vi "Heat2D_Solver.vi"(0 "F(t, x, y)":dbl[][][](array[numeric]), 1 "Initial Value":dbl[][](array[numeric]), 5 "k":dbl=1.0, 7 "a":dbl, 9 "Domain":T1={"t"={"initial t"=0.0, "final t"=1.0, "# of t-points"=11}, "x"={"start x"=0.0, "end x"=1.0, "# of x-points"=11}, "y"={"start y"=0.0, "end y"=1.0, "# of y-points"=11}}, 11 "error in (no error)":errorcluster, 12 "Boundary Condition":cluster{"type":T2, "Value":dbl[][]}[](array[cluster]) {"type" items=["Dirichlet", "Neumann"]}) -> (4 "U(t, x, y)":dbl[][][](array[numeric]), 15 "error out":errorcluster)   [LabVIEW 2020, in "NI_PDE.lvlib"]
uses:
  <vilib>/gmath/NI_PDE.lvlib
  <vilib>/gmath/pde.llb/Common/PDE_BC Type.ctl
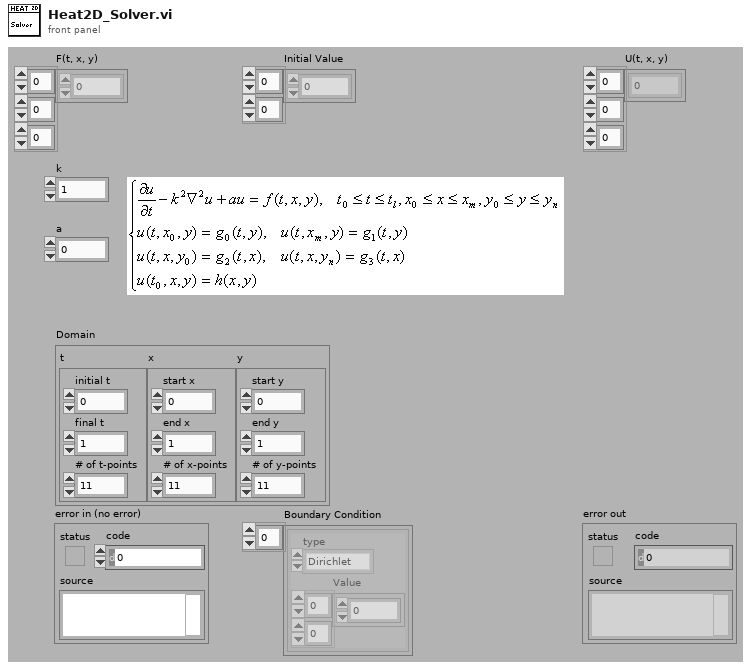
[diagram p1: front panel]
types:
  T1 = cluster{"t":cluster{"initial t":dbl, "final t":dbl, "# of t-points":i32}, "x":cluster{"start x":dbl, "end x":dbl, "# of x-points":i32}, "y":cluster{"start y":dbl, "end y":dbl, "# of y-points":i32}}
  T2 = typedef "NI_PDE.lvlib/PDE_BC Type.ctl" = i32
  T3 = cluster{"rx":dbl, "ry":dbl, "s":dbl, "c":dbl, "deltaT":dbl, "deltaX":dbl, "deltaY":dbl}
  T4 = cluster{"X LU Factor":cluster{"L":dbl[], "U":cluster{"Diagonal":dbl[], "Super Diagonal":dbl[], "2nd Super Diagonal":dbl[]}, "Pivot":i32[]}, "Y LU Factor":cluster{"L":dbl[], "U":cluster{"Diagonal":dbl[], "Super Diagonal":dbl[], "2nd Super Diagonal":dbl[]}, "Pivot":i32[]}, "X Tridiagonal":cluster{"SubDiagonal":dbl[], "MainDiagonal":dbl[], "SuperDiagonal":dbl[]}, "Y Tridiagonal":cluster{"SubDiagonal":dbl[], "MainDiagonal":dbl[], "SuperDiagonal":dbl[]}}
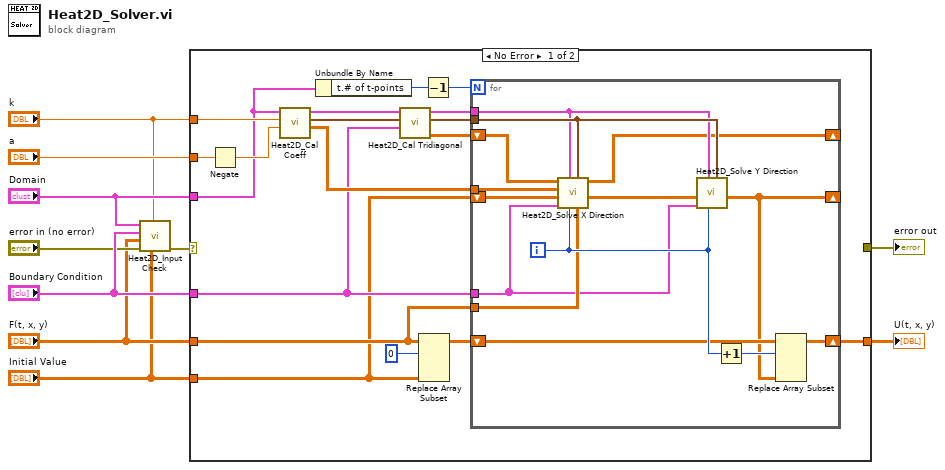
[diagram p0: block diagram]
diagram:
  n1 = call <vilib>:"Heat2D_Input Check.vi"("Initial Value"="Initial Value", "k"="k", "error in (no error)"="error in (no error)", "F(t, x, y)"="F(t, x, y)", "Boundary Condition"="Boundary Condition", "Domain"="Domain") -> ("error out"=w7:errorcluster)  [unwired: 5 out]
  n2 = case shown="No Error" w7 {
    selector: w7 -> [_ w43]
    tunnel: "k" -> [w28 _]
    tunnel: "a" -> [w27 _]
    tunnel: "Initial Value" -> [w11 _]
    tunnel: "Boundary Condition" -> [w12 _]
    tunnel: "F(t, x, y)" -> [w13 _]
    tunnel: "Domain" -> [w14 _]
    tunnel: [_ w43] -> w3
    tunnel: [w20 _] -> w2
    frame No Error {
      n3 = Negate(x=w27) -> (-x=w24:dbl)
      n4 = call <vilib>:"Heat2D_Cal Coeff.vi"("a"=w24, "k"=w28, "Domain"=w14) -> ("Matr_RHS"=w23:dbl[][], "Coefficients"=w17:T3, "Domain Dup"=w26:T1)  [unwired: 6 out]
      n5 = Unbundle By Name(w14) -> ("t.# of t-points"=w16:i32)
      n6 = call <vilib>:"Heat2D_Cal Tridiagonal.vi"("Boundary Condition"=w12, "Coefficients"=w17, "Domain"=w26) -> ("X RHS"=w18:dbl[][], "Coefficients Dup"=w25:T3, "TriDia Cluster"=w19:T4)  [unwired: 1 in, 5 out]
      n7 = Replace Array Subset(array=w13, new element=w11, index (dim 0)=0 ("index (page)")) -> (w22:dbl[][][])  [unwired: 2 in]
      n8 = Decrement(x=w16) -> (x-1=w15:i32)
      n9 = for {
        N: w15 -> [_]
        shift-right: [w29] -> _
        shift-left: w11 -> [w32]
        tunnel: w25 -> [w42]
        tunnel: w12 -> [w31]
        tunnel: w13 -> [w34]
        tunnel: w23 -> [w33]
        shift-right: [w35] -> w20
        shift-left: w22 -> [w36]
        tunnel: w19 -> [w40]
        shift-right: [w38] -> _
        shift-left: w18 -> [w39]
        i -> [w41]
        n10 = call <vilib>:"Heat2D_Solve X Direction.vi"("F(t, x, y)"=w34, "Coefficients"=w42, "step"=w41, "TriDia Cluster"=w40, "Boundary Condition"=w31, "U(n)"=w32, "Matr_RHS"=w33, "X RHS"=w39) -> ("U(n+1/2)"=w30:dbl[][], "X RHS out"=w38:dbl[][])  [unwired: 2 out]
        n11 = call <vilib>:"Heat2D_Solve Y Direction.vi"("Coefficients"=w42, "step"=w41, "TriDia Cluster"=w40, "Boundary Condition"=w31, "U(n+1/2)"=w30) -> ("U(n+1)"=w29:dbl[][])  [unwired: 2 in, 4 out]
        n12 = Increment(x=w41) -> (x+1=w37:i32)
        n13 = Replace Array Subset(array=w36, new element=w29, index (dim 0)=w37) -> (w35:dbl[][][])  [unwired: 2 in]
      }
    }
    frame Error {
    }
  }
  "error out" <- w3
  "U(t, x, y)" <- w2
